vi "4to2line decoder.vi"() -> ()   [LabVIEW 2009]
panel:
  out "Boolean 6":bool
  out "Boolean 5":bool
  out "Boolean 4":bool
  out "Boolean 3":bool
  in  "Boolean 2":bool
  in  "Boolean":bool
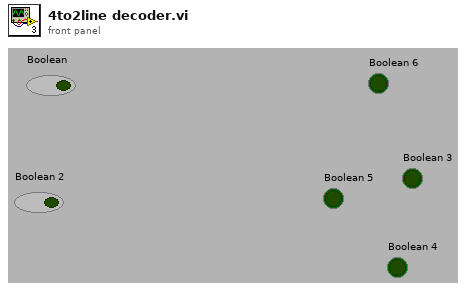
[diagram p1: front panel]
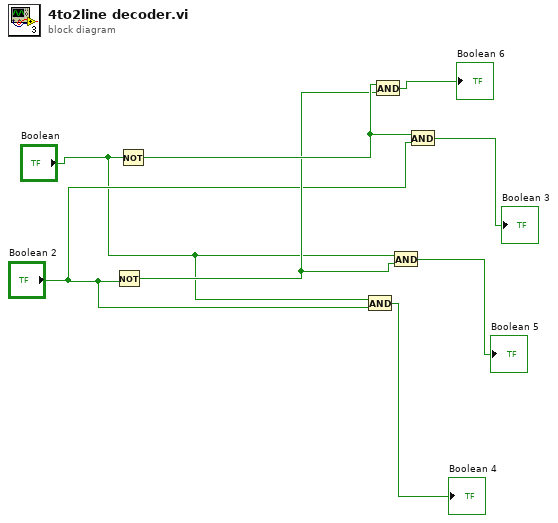
[diagram p0: block diagram]
diagram:
  n1 = Not(x="Boolean 2") -> (.not. x?=w5:bool)
  n2 = Not(x="Boolean") -> (.not. x?=w7:bool)
  n3 = And(x="Boolean", y="Boolean 2") -> (x .and. y?=→"Boolean 4":bool)
  n4 = And(x=w7, y=w5) -> (x .and. y?=→"Boolean 6":bool)
  n5 = And(x="Boolean", y=w5) -> (x .and. y?=→"Boolean 5":bool)
  n6 = And(x=w7, y="Boolean 2") -> (x .and. y?=→"Boolean 3":bool)
